vi "max-number.vi"() -> ()   [LabVIEW 2011]
panel:
  out "V":dbl[unit]
  out "static_presure":dbl[unit]
  out "static_temperature":dbl[unit]
  in  "M":dbl
  in  "altitude":dbl[unit]
  out "total-temperature":dbl[unit]
  out "total-pressure":dbl[unit]
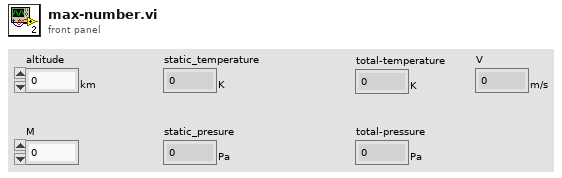
[diagram p1: front panel]
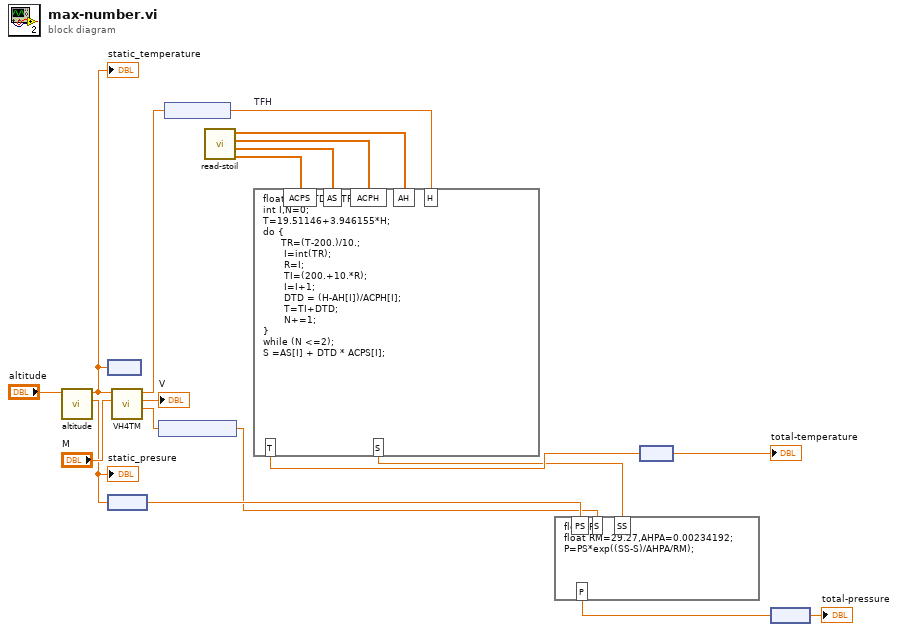
[diagram p0: block diagram]
diagram:
  n1 = call "altitude.vi"("altitude"="altitude") -> ("presure"=w6:dbl[unit], "temperature"=w15:dbl[unit])  [unwired: 9 in]
  "static_temperature" <- w15
  "static_presure" <- w6
  n2 = node(w15) -> ()  [unwired: 1 out]
  n3 = node(w6) -> (w5:dbl)
  n4 = call "VH4TM.vi"("M"="M", "T"=w15) -> ("S"=w4:dbl[unit], "V"=→"V":dbl[unit], "H"=w17:dbl[unit])  [unwired: 7 in]
  n5 = node(w4) -> (w3:dbl)
  n6 = node(w17) -> (w14:dbl)
  n7 = call "read-stoil.vi"() -> ("ACPS"=w12:dbl[], "AS"=w13:dbl[], "ACPH"=w11:dbl[], "AH"=w10:dbl[])  [unwired: 8 in]
  n8 = formula code="float T,S,DTD,TI,TR,R;\nint I,N=0;\nT=19.51146+3.946155*H;\ndo {\n      TR=(T-200.)/10.;\n       I=int(TR);\n       R=I;\n       TI=(200.+10.*R);\n       I=I+1;\n       DTD = (H-AH[I])/ACPH[I];\n       T=TI+DTD;\n       N+=1;\n}\nwhile (N <=2);\nS =AS[I] + DTD * ACPS[I];" "TFH"("H"=w14, "AS"=w13, "ACPS"=w12, "AH"=w10, "ACPH"=w11) -> ("T"=w9:dbl, "S"=w2:dbl)
  n9 = formula code="float P;\nfloat RM=29.27,AHPA=0.00234192;\nP=PS*exp((SS-S)/AHPA/RM);"("PS"=w5, "S"=w3, "SS"=w2) -> ("P"=w7:dbl)
  n10 = node(w9) -> (→"total-temperature":dbl[unit])
  n11 = node(w7) -> (→"total-pressure":dbl[unit])
